vi "init.vi"(8 "error in (no error)":errorcluster, 10 "configDirectoryPathWindows":path, 11 "LoopTimer in":refnum<class "LoopTimer.lvclass">) -> (0 "error out":errorcluster, 3 "LoopTimer out":refnum<class "LoopTimer.lvclass">)   [LabVIEW 2013, in "ComponentData.lvlib" / "LoopTimer.lvclass"]
uses:
  <userlib>/Common/Component/Application/RT/ComponentData/LoopTimer/LoopTimer.lvclass
  <userlib>/Common/Component/Application/RT/ComponentData/LoopTimer/LoopTimer.lvclass/LoopTimer.ctl
  <userlib>/Common/Component/Application/RT/ComponentData/ConfigurationHandler/LoopConfig/LoopConfig.lvclass
  <userlib>/Common/Component/Application/RT/ComponentData/ConfigurationHandler/LoopInternalConfig/LoopInternalConfig.lvclass
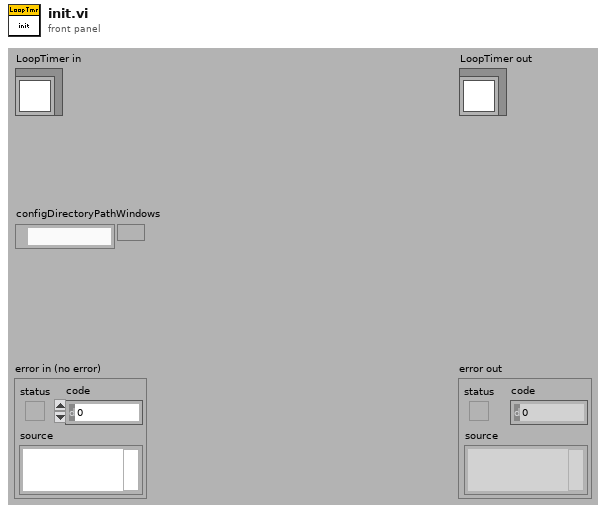
[diagram p1: front panel]
types:
  T1 = enum32{"invalid OS target", "Mac OS", "Windows 3.1", "Windows 95/NT", "Solaris 1", "Solaris 2", "HP-UX", "PowerMAX", "Linux", "Irix", "Rhapsody", "BeOS", "AIX", "OSF1", "VxWorks", "PharLap", "Carbon", "RTX", "Windows x64", "Linux x64"}
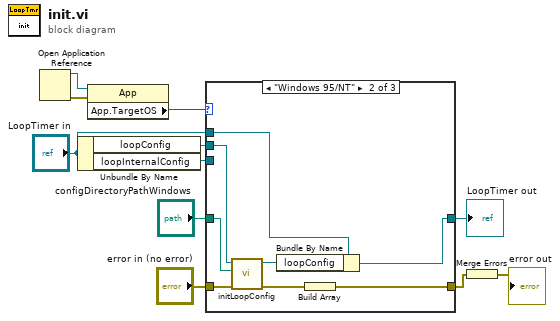
[diagram p0: block diagram]
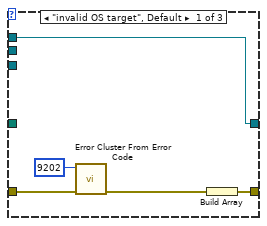
[diagram p2: hidden frame]
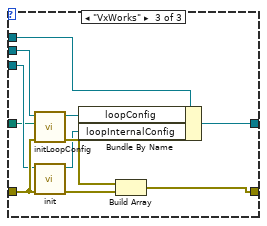
[diagram p3: hidden frame]
diagram:
  n1 = Open Application Reference() -> (0:w2:errorcluster, 3:w3:refnum<vi>)  [unwired: 4 in]
  n2 = Unbundle By Name("LoopTimer in") -> ("loopConfig"=w7:refnum<class "LoopConfig.lvclass">, "loopInternalConfig"=w6:refnum<class "LoopInternalConfig.lvclass">)
  n3 = property class="App"(reference=w3, error in=w2) -> ("App.TargetOS"=w1:T1)  [unwired: 2 out]
  n4 = case shown="\"Windows 95/NT\"" w1 {
    tunnel: "error in (no error)" -> [w15 w24 w35]
    tunnel: "LoopTimer in" -> [w12 w23 w34]
    tunnel: [w12 w22 w33] -> w8
    tunnel: w7 -> [_ w21 w32]
    tunnel: w6 -> [_ _ w31]
    tunnel: [w13 w19 w28] -> w5
    tunnel: "configDirectoryPathWindows" -> [_ w18 w27]
    frame "invalid OS target", Default {
      n5 = call <vilib>:"Error Cluster From Error Code.vi"("error in (no error)"=w15, "error code (0)"=9202) -> ("error out"=w14:errorcluster)  [unwired: 7 in]
      n6 = Build Array(w14) -> (w13:errorcluster[])
    }
    frame "Windows 95/NT" {
      n7 = call <userlib>:"initLoopConfig.vi"("error in (no error)"=w24, "configDirectoryPathWindows"=w18, "LoopConfig in"=w21) -> ("error out"=w20:errorcluster, "LoopConfig out"=w17:refnum<class "LoopConfig.lvclass">)  [unwired: 7 in]
      n8 = Bundle By Name(cluster=w23, "loopConfig"=w17) -> (w22:refnum<class "LoopTimer.lvclass">)
      n9 = Build Array(w20) -> (w19:errorcluster[])
    }
    frame "VxWorks" {
      n10 = call <userlib>:"initLoopConfig.vi"("error in (no error)"=w35, "configDirectoryPathWindows"=w27, "LoopConfig in"=w32) -> ("error out"=w30:errorcluster, "LoopConfig out"=w26:refnum<class "LoopConfig.lvclass">)  [unwired: 7 in]
      n11 = call <userlib>:"init.vi"("error in (no error)"=w35, "LoopInternalConfig in"=w31) -> ("error out"=w29:errorcluster, "LoopInternalConfig out"=w25:refnum<class "LoopInternalConfig.lvclass">)  [unwired: 8 in]
      n12 = Bundle By Name(cluster=w34, "loopConfig"=w26, "loopInternalConfig"=w25) -> (w33:refnum<class "LoopTimer.lvclass">)
      n13 = Build Array(w30, w29) -> (w28:errorcluster[])
    }
  }
  "LoopTimer out" <- w8
  n14 = Merge Errors(w5) -> (→"error out":errorcluster)
